vi "prepareCmdStatus.vi"(8 "error in (no error)":errorcluster, 9 "cmdStatus":string(combo)="ack", 10 "packetConnID":T1, 11 "tcpServer in":refnum<class "TcpServer.lvclass">) -> (0 "error out":errorcluster, 3 "tcpServer out":refnum<class "TcpServer.lvclass">)   [LabVIEW 2018, in "TcpServer.lvclass"]
doc: "Prepare cmd Status."
uses:
  TcpServer.lvclass
  typedef/packetConnIDTypeDef.ctl
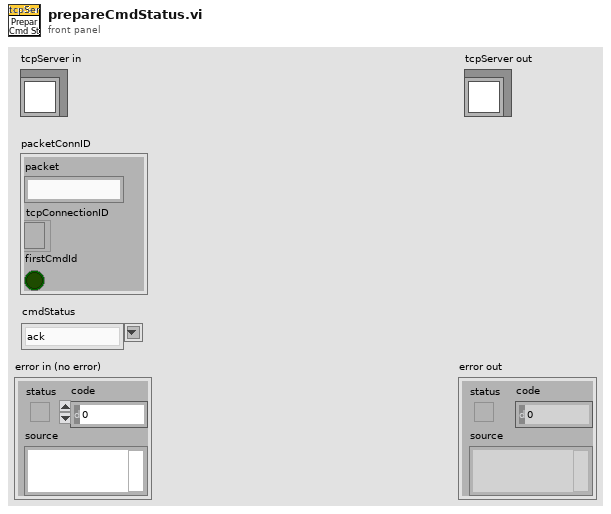
[diagram p1: front panel]
types:
  T1 = typedef "TcpServer.lvclass/packetConnIDTypeDef.ctl" = cluster{"packet":string, "tcpConnectionID":refnum<k5>, "firstCmdId":bool}
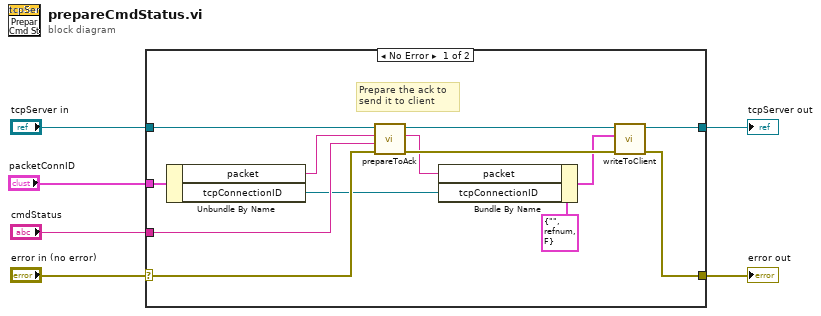
[diagram p0: block diagram]
diagram:
  n1 = case shown="No Error" "error in (no error)" {
    selector: "error in (no error)" -> [w15 w21]
    tunnel: [w18 w21] -> w5
    tunnel: [w19 w20] -> w3
    tunnel: "tcpServer in" -> [w17 w20]
    tunnel: "cmdStatus" -> [w13 _]
    tunnel: "packetConnID" -> [w9 _]
    frame No Error {
      # "Prepare the ack to\nsend it to client"
      n2 = Unbundle By Name(w9) -> ("packet"=w8:string, "tcpConnectionID"=w7:refnum<k5>)
      n3 = call "prepareToAck.vi"("error in (no error)"=w15, "cmdStatus"=w13, "cmd"=w8, "TcpServer in"=w17) -> ("error out"=w14:errorcluster, "JSON string"=w11:string, "TcpServer out"=w16:refnum<class "TcpServer.lvclass">)  [unwired: 5 in]
      n4 = Bundle By Name(cluster=T1 {"packet"="", "tcpConnectionID"=refnum, "firstCmdId"=FALSE} ("packetConnID"), "packet"=w11, "tcpConnectionID"=w7) -> (w10:T1)
      n5 = call "writeToClient.vi"("error in (no error)"=w14, "packetConnID"=w10, "tcpServer in"=w16) -> ("error out"=w18:errorcluster, "tcpServer out"=w19:refnum<class "TcpServer.lvclass">)  [unwired: 7 in]
    }
    frame Error {
    }
  }
  "error out" <- w5
  "tcpServer out" <- w3
